vi "setGlobals0.vi"() -> ()   [LabVIEW 2011]
panel:
  in  "Ring":u16(ring)
  in  "MFCs":T1 {"ALMFC1 5"."MFC Range" items=["0-10 sccm", "0-100 sccm", "0-1000 sccm"]; "ALMFC1 4"."MFC Range" items=["0-10 sccm", "0-100 sccm", "0-1000 sccm"]; "ALMFC1 3"."MFC Range" items=["0-10 sccm", "0-100 sccm", "0-1000 sccm"]; "ALMFC1 2"."MFC Range" items=["0-10 sccm", "0-100 sccm", "0-1000 sccm"]; "ALMFC1"."MFC Range" items=["0-10 sccm", "0-100 sccm", "0-1000 sccm"]; "HMFC1"."MFC Range" items=["0-10 sccm", "0-100 sccm", "0-1000 sccm"]; "NMFC1"."MFC Range" items=["0-10 sccm", "0-100 sccm", "0-1000 sccm"]}
  in  "Card 1":T2 caption="Card 1 Channels" {"Channel 4" items=["N2 flow (NMFC1)", "H2 flow (HMFC1)", "Al flow (AlMFC1)"]; "Channel 3" items=["N2 flow (NMFC1)", "H2 flow (HMFC1)", "Al flow (AlMFC1)"]; "Channel 2" items=["N2 flow (NMFC1)", "H2 flow (HMFC1)", "Al flow (AlMFC1)"]; "Channel 1" items=["N2 flow (NMFC1)", "H2 flow (HMFC1)", "Al flow (AlMFC1)"]}
  out "output array":string[](array[string])
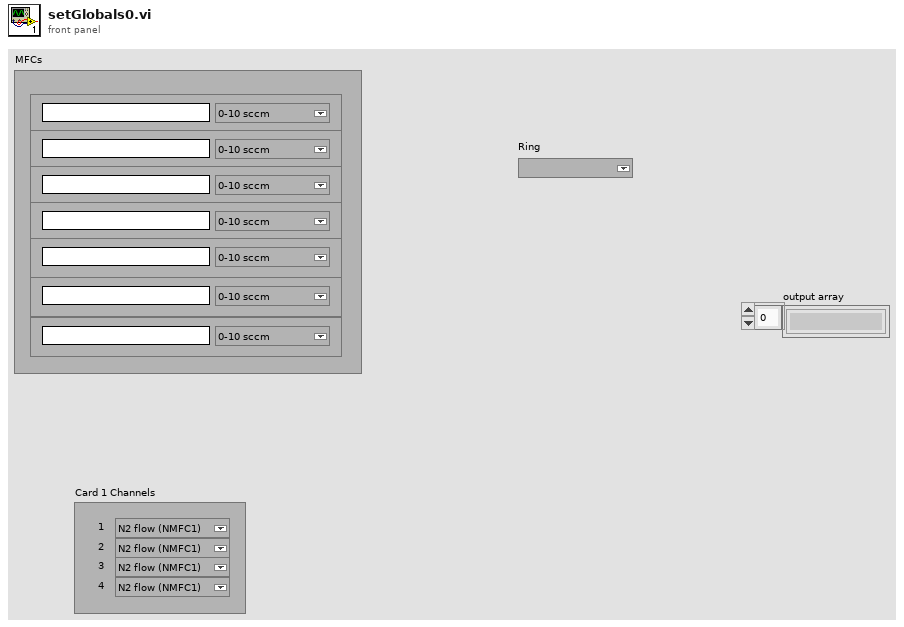
[diagram p1: front panel]
types:
  T1 = cluster{"NMFC1":cluster{"MFC Range":u16, "MFC Name":string}, "HMFC1":cluster{"MFC Range":u16, "MFC Name":string}, "ALMFC1":cluster{"MFC Range":u16, "MFC Name":string}, "ALMFC1 2":cluster{"MFC Range":u16, "MFC Name":string}, "ALMFC1 3":cluster{"MFC Range":u16, "MFC Name":string}, "ALMFC1 4":cluster{"MFC Range":u16, "MFC Name":string}, "ALMFC1 5":cluster{"MFC Range":u16, "MFC Name":string}}
  T2 = cluster{"Channel 1":u16, "Channel 2":u16, "Channel 3":u16, "Channel 4":u16}
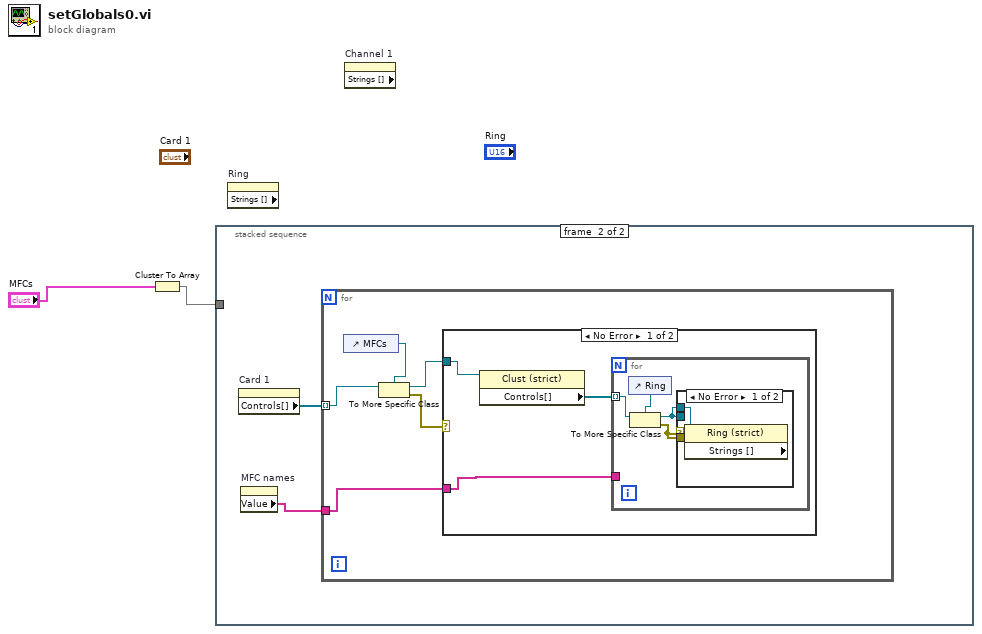
[diagram p0: block diagram]
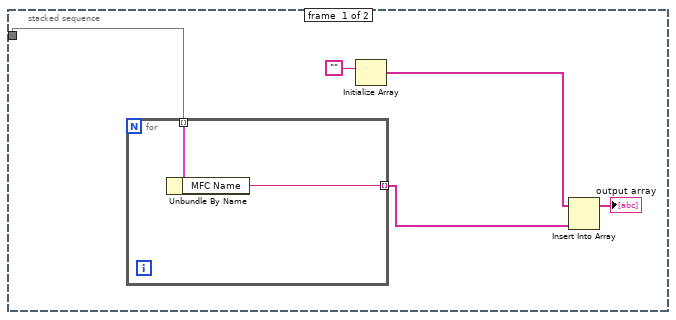
[diagram p2: hidden frame]
diagram:
  n1 = Cluster To Array(cluster="MFCs") -> (array=w2:cluster{"MFC Range":u16, "MFC Name":string}[])
  n2 = stacked-sequence {
    tunnel: w2 -> [w4 _]
    frame #0 {
      n3 = for {
        tunnel: w4 -> [w9] mode=indexing
        tunnel: [w8] -> w6 mode=indexing
        n4 = Unbundle By Name(w9) -> ("MFC Name"=w8:string)
      }
      n5 = Initialize Array("") -> (w5:string[])  [unwired: 1 in]
      n6 = Insert Into Array(array=w5, new element=w6) -> (→"output array":string[])  [unwired: 1 in]
    }
    frame #1 {
      n7 = property on="Card 1" class="Clust (strict)"() -> ("Controls[]"=w11:refnum<vi>[])  [unwired: 2 in, 2 out]
      n8 = property on="MFC names" class="Arr (strict)"() -> ("Value"=w10:string[])  [unwired: 2 in, 2 out]
      n9 = for {
        tunnel: w11 -> [w14] mode=indexing
        tunnel: w10 -> [w13]
        n10 = control-ref of="MFCs"() -> (w12:refnum<vi>)
        n11 = To More Specific Class(target class=w12, reference=w14) -> (specific class reference=w15:refnum<vi>, error out=w16:errorcluster)  [unwired: 1 in]
        n12 = case shown="No Error" w16 {
          tunnel: w15 -> [w18 _]
          tunnel: w13 -> [w19 _]
          frame No Error {
            n13 = property class="Clust (strict)"(reference=w18) -> ("Controls[]"=w17:refnum<vi>[])  [unwired: 1 in, 2 out]
            n14 = for {
              tunnel: w19 -> [_]
              tunnel: w17 -> [w23] mode=indexing
              n15 = control-ref of="Ring"() -> (w22:refnum<vi>)
              n16 = To More Specific Class(target class=w22, reference=w23) -> (specific class reference=w21:refnum<vi>, error out=w20:errorcluster)  [unwired: 1 in]
              n17 = case shown="No Error" w20 {
                tunnel: w21 -> [_ _]
                tunnel: w21 -> [w25 _]
                tunnel: w20 -> [w24 _]
                frame No Error {
                  n18 = property class="Ring (strict)" props=["Strings []"](reference=w25, error in=w24) -> ()  [unwired: 3 out]
                }
                frame Error {
                }
              }
            }
          }
          frame Error {
          }
        }
      }
    }
  }
  n19 = property on="Ring" class="Ring (strict)" props=["Strings []"]() -> ()  [unwired: 2 in, 3 out]
  n20 = property on="Channel 1" class="Ring (strict)" props=["Strings []"]() -> ()  [unwired: 2 in, 3 out]
